vi "set_double_check_moving.vi"(8 "error in (no error)":errorcluster, 10 "double check moving":cluster{"1st check":bool, "2nd check":bool}[](array[cluster]), 11 "MotorSystem in":refnum<class "MotorSystem.lvclass">) -> (0 "error out":errorcluster, 3 "MotorSystem out":refnum<class "MotorSystem.lvclass">)   [LabVIEW 2016, in "MotionControl.lvlib" / "MotorSystem.lvclass"]
uses:
  <userlib>/MotionControl/MotorSystem/MotorSystem.lvclass
  <userlib>/MotionControl/MotorSystem/MotorSystem.lvclass/MotorSystem.ctl
  <userlib>/MotionControl/OneMotion/OneMotion.lvclass/OneMotion.ctl
  <userlib>/MotionControl/StepMotor/StepMotor.lvclass/StepMotor.ctl
  <userlib>/MotionControl/MotorSystem/get_motions.vi
  <userlib>/MotionControl/StepMotor/set_moving.vi
  <userlib>/MotionControl/OneMotion/get_StepMotor.vi
  <userlib>/MotionControl/OneMotion/set_StepMotor.vi
  <userlib>/MotionControl/MotorSystem/set_motions.vi
  <userlib>/MotionControl/StepMotor/StepMotor.lvclass
  <userlib>/MotionControl/OneMotion/OneMotion.lvclass
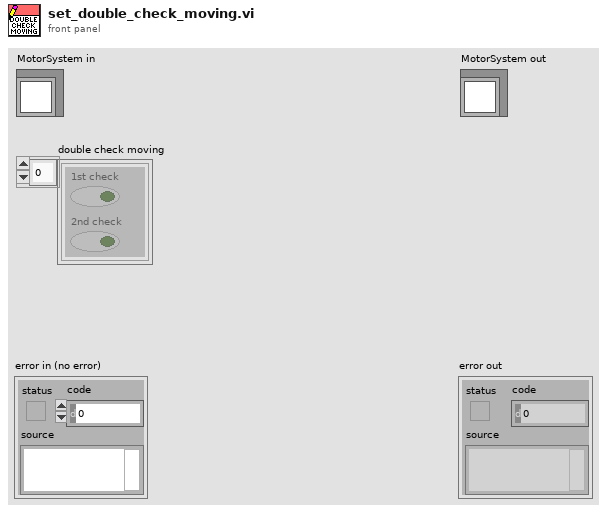
[diagram p1: front panel]
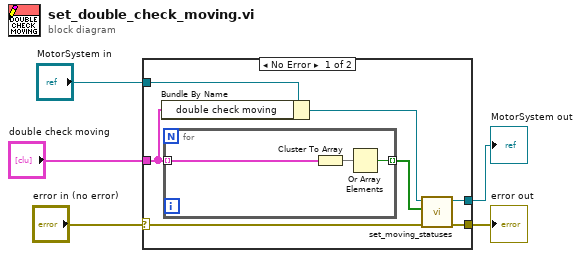
[diagram p0: block diagram]
diagram:
  n1 = case shown="No Error" "error in (no error)" {
    selector: "error in (no error)" -> [w7 w16]
    tunnel: [w6 w16] -> w4
    tunnel: [w10 w17] -> w2
    tunnel: "MotorSystem in" -> [w12 w17]
    tunnel: "double check moving" -> [w9 _]
    frame No Error {
      n2 = Bundle By Name(cluster=w12, "double check moving"=w9) -> (w11:refnum<class "MotorSystem.lvclass">)
      n3 = for {
        tunnel: w9 -> [w15] mode=indexing
        tunnel: [w13] -> w8 mode=indexing
        n4 = Cluster To Array(cluster=w15) -> (array=w14:bool[])
        n5 = Or Array Elements(Boolean array=w14) -> (logical OR=w13:bool)
      }
      n6 = call <userlib>:"set_moving_statuses.vi"("error in (no error)"=w7, "moving statuses"=w8, "MotorSystem输入"=w11) -> ("error out"=w6:errorcluster, "MotorSystem输出"=w10:refnum<class "MotorSystem.lvclass">)  [unwired: 7 in]
    }
    frame Error {
    }
  }
  "error out" <- w4
  "MotorSystem out" <- w2
